vi "GenINI_Wire_Terminal.vi"(8 "error in":errorcluster, 9 "Terminal  name":string, 10 "Wire source ref":refnum<vi>, 11 "vi ref":refnum<vi>) -> (0 "error out":errorcluster, 2 "Wire source ref dup":refnum<vi>, 3 "vi ref dup":refnum<vi>)   [LabVIEW 2009]
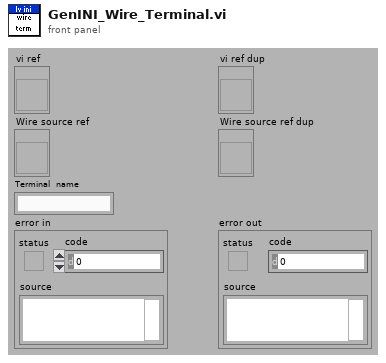
[diagram p1: front panel]
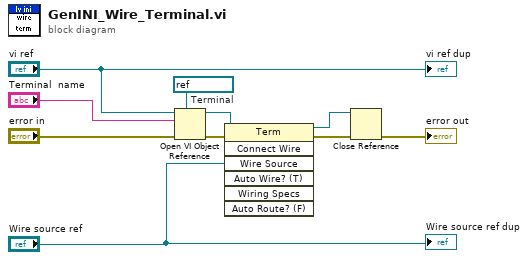
[diagram p0: block diagram]
diagram:
  w10 = refnum<vi> refnum  # Terminal
  n1 = Open VI Object Reference(7:w10, 8:"error in", 10:"Terminal  name", 11:"vi ref") -> (0:w8:errorcluster, 3:w5:refnum<vi>)
  n2 = invoke class="Term" method="Connect Wire"(reference=w5, error in=w8, "Wire Source"="Wire source ref") -> (reference out=w1:refnum<vi>, error out=w3:errorcluster)  [unwired: 4 in, 5 out]
  n3 = Close Reference(reference=w1, error in (no error)=w3) -> (error out=→"error out":errorcluster)
  "Wire source ref dup" <- "Wire source ref"
  "vi ref dup" <- "vi ref"
